vi "Main.vi"() -> ()   [LabVIEW 2018]
uses:
  LoadCellType.ctl
  MotorUnits.ctl
  <vilib>/Analysis/baseanly.llb/Mean (DBL).vi
  <vilib>/FPGAPlugInAG/myRIO-1900/niLvFpga_Open_myRIO-1900.vi
  <vilib>/rvi/interface/common/dynamic/niFpgaDynamicAddResources.vi
  <vilib>/FPGAPlugInAG/Dynamic/niLvFpga_Run_Dynamic.vi
  <vilib>/Utility/error.llb/Error Cluster From Error Code.vi
  <vilib>/rvi/errors/niLvFpgaAdjustHostInterfaceError.vi
  <vilib>/FPGAPlugInAG/Dynamic/niLvFpga_Abort_Dynamic.vi
  <vilib>/FPGAPlugInAG/Dynamic/niLvFpga_Close_Dynamic.vi
  <vilib>/rvi/interface/nirviOpenFPGA/nirviOpenFPGA.xnode
  FPGA Bitfiles/StandProgram_FPGATarget3_FPGARightReadout_3aa7no0+bKE.lvbitx
  FPGARightReadout.vi
  <vilib>/rvi/interface/nirviMethod/nirviMethod.xnode
  <vilib>/rvi/interface/nirviReadWriteControl/nirviReadWriteControl.xnode
  <vilib>/rvi/interface/nirviCloseFPGA/nirviCloseFPGA.xnode
  FPGA Bitfiles/StandProgram_FPGATarget_FPGACentreReadou_e9s0Pr-w3KU.lvbitx
  FPGACentreReadout.vi
  FPGA Bitfiles/StandProgram_FPGATarget2_FPGALeftReadout_XaESxvNjBQc.lvbitx
  FPGALeftReadout.vi
  NiFpgaLv.dll
  <vilib>/rvi/interface/Simulation/niFpgaSimulationCallBeginRW.vi
  <vilib>/Analysis/NI_AALBase.lvlib
  <userlib>/dxl_x86_c/dxl_x86_c.lvlib
panel:
  in  "Motor 2 Operating Mode":u16(ring)=5 caption="Operating Mode" items=["Please Select", "Current Control", "Velocity", "Position", "Extended Position", "Current-based Position Control"]
  out "Current Motor 1 Position":dbl(knob) scale=0.0..360.0
  in  "Motor 1 Operating Mode":u16(ring)=5 caption="Operating Mode" items=["Please Select", "Current Control", "Velocity", "Position", "Extended Position", "Current-based Position Control"]
  out "function return":i32
  in  "Left Stand":enum32{"Main", "Setup"}(tab)
  out "Left Motor Frequency":dbl caption="Motor Frequency"
  in  "Left PWM frequency":i16=50 caption="PWM Frequency (Hz)" min=50 max=400
  in  "Left PWM Switch":bool caption="PWM Switch"
  in  "Left PWM pulse width":u32=1000 caption="PWM Length (us)" min=1000 max=2000
  out "Left Current":dbl(knob) caption="Current (A)" scale=0.0..90.0
  out "Left Voltage":dbl(knob) caption="Voltage (V)" scale=0.0..60.0
  out "Left LC1":dbl(slide) scale=-10.0..10.0
  out "Left LC2":dbl(slide) scale=-5.0..5.0
  out "Left LC3":dbl(slide) scale=-5.0..5.0
  in  "Left Motor Units":T1 caption="Units" items=["RPM", "Hz"]
  out "Left LC1 Reading":i32 caption="Reading"
  in  "Left LC3 Calibrate":bool
  in  "Left LC3 Calibration Weight (kg)":dbl caption="Calibration Weight (kg)"
  in  "Left LC3 Type":T2 caption="Load Cell Type" items=["5kg", "10kg", "50kg"]
  out "Left LC3 zero point":i32 caption="Zero Point"
  in  "Left LC3 Tare":bool
  in  "Left LC2 Calibrate":bool
  in  "Left LC2 Calibration Weight (kg)":dbl caption="Calibration Weight (kg)"
  in  "Left LC2 Type":T2 caption="Load Cell Type" items=["5kg", "10kg", "50kg"]
  out "Left LC2 zero point":i32 caption="Zero Point"
  in  "Left LC2 Tare":bool
  in  "Left LC1 Calibrate 3":bool
  in  "Left LC1 Calibration Weight (kg)":dbl caption="Calibration Weight (kg)"
  in  "Left LC1 Type":T2=1 caption="Load Cell Type" items=["5kg", "10kg", "50kg"]
  out "Left LC1 zero point":i32=34722 caption="Zero Point"
  in  "Left LC1 Tare 3":bool
  out "Left LC3 Reading":i32 caption="Reading"
  out "Left LC2 Reading":i32 caption="Reading"
  in  "Left Resistance non-Vout (Ohms)":dbl=13.81
  in  "Left Resistance Vout (Ohms)":dbl=1.642
  out "Left Raw Load Cell Readings":cluster{"Data":i32, "Data 2":i32, "Data 3":i32}(graph) caption="Raw Load Cell Readings"
  out "Left LC3 Calibration Constant":dbl format="%#_13g"
  out "Left LC2 Calibration Constant":dbl format="%#_13g"
  out "Left LC1 Calibration Constant":dbl format="%#_13g"
  in  "Centre Stand":enum32{"Main", "Setup"}(tab)
  out "Right LC1":dbl(slide) scale=-10.0..10.0
  out "Left LC2":dbl(slide) scale=-10.0..10.0
  out "Centre LC3":dbl(slide) scale=-10.0..10.0
  out "Centre LC1 Reading":i32 caption="Reading"
  in  "Centre LC3 Calibrate":bool
  in  "Centre LC3 Calibration Weight (kg)":dbl caption="Calibration Weight (kg)"
  in  "Centre LC3 Type":T2=1 caption="Load Cell Type" items=["5kg", "10kg", "50kg"]
  out "Centre LC3 zero point":i32 caption="Zero Point"
  in  "Centre LC3 Tare":bool
  in  "Centre LC2 Calibrate":bool
  in  "Centre LC2 Calibration Weight (kg)":dbl caption="Calibration Weight (kg)"
  in  "Centre LC2 Type":T2=1 caption="Load Cell Type" items=["5kg", "10kg", "50kg"]
  out "Centre LC2 zero point":i32 caption="Zero Point"
  in  "Centre LC2 Tare":bool
  in  "Centre LC1 Calibrate":bool
  in  "Centre LC1 Calibration Weight (kg)":dbl caption="Calibration Weight (kg)"
  in  "Centre LC1 Type":T2=1 caption="Load Cell Type" items=["5kg", "10kg", "50kg"]
  out "Centre LC1 zero point":i32=34722 caption="Zero Point"
  in  "Centre LC1 Tare":bool
  out "Centre LC3 Reading":i32 caption="Reading"
  out "Centre LC2 Reading":i32 caption="Reading"
  out "Centre Raw Load Cell Readings":cluster{"Data":i32, "Data 2":i32, "Data 3":i32}(graph) caption="Raw Load Cell Readings"
  out "Centre LC3 Calibration Constant":dbl format="%#_13g"
  out "Centre LC2 Calibration Constant":dbl format="%#_13g"
  out "Centre LC1 Calibration Constant":dbl format="%#_13g"
  out "StopLoops":bool
  in  "Program Stop":bool
  out "Current Motor 2 Position":dbl(knob) scale=0.0..360.0
  in  "Target Motor 2 Position":dbl(knob) scale=0.0..360.0
  in  "Target Motor 1 Position":dbl(knob) scale=0.0..360.0
  in  "Right Stand":enum32{"Main", "Setup"}(tab)
  out "Right Motor Frequency":dbl caption="Motor Frequency"
  in  "Right PWM frequency":i16=50 caption="PWM Frequency (Hz)" min=50 max=400
  in  "Right PWM Switch":bool caption="PWM Switch"
  in  "Right PWM pulse width":u32=1000 caption="PWM Length (us)" min=1000 max=2000
  out "Right Current":dbl(knob) caption="Current (A)" scale=0.0..90.0
  out "Right Voltage":dbl(knob) caption="Voltage (V)" scale=0.0..60.0
  out "Right LC1":dbl(slide) scale=-10.0..10.0
  out "Right LC2":dbl(slide) scale=-5.0..5.0
  out "Right LC3":dbl(slide) scale=-5.0..5.0
  in  "Right Motor Units":T1 caption="Units" items=["RPM", "Hz"]
  out "Right LC1 Reading":i32 caption="Reading"
  in  "Right LC3 Calibrate":bool
  in  "Right LC3 Calibration Weight (kg)":dbl caption="Calibration Weight (kg)"
  in  "Right LC3 Type":T2 caption="Load Cell Type" items=["5kg", "10kg", "50kg"]
  out "Right LC3 zero point":i32 caption="Zero Point"
  in  "Right LC3 Tare":bool
  in  "Right LC2 Calibrate":bool
  in  "Right LC2 Calibration Weight (kg)":dbl caption="Calibration Weight (kg)"
  in  "Right LC2 Type":T2 caption="Load Cell Type" items=["5kg", "10kg", "50kg"]
  out "Right LC2 zero point":i32 caption="Zero Point"
  in  "Right LC2 Tare":bool
  in  "Right LC1 Calibrate":bool
  in  "Right LC1 Calibration Weight (kg)":dbl caption="Calibration Weight (kg)"
  in  "Right LC1 Type":T2=1 caption="Load Cell Type" items=["5kg", "10kg", "50kg"]
  out "Right LC1 zero point":i32=34722 caption="Zero Point"
  in  "Right LC1 Tare":bool
  out "Right LC3 Reading":i32 caption="Reading"
  out "Right LC2 Reading":i32 caption="Reading"
  in  "Right Resistance non-Vout (Ohms)":dbl=13.81
  in  "Right Resistance Vout (Ohms)":dbl=1.642
  out "Right Raw Load Cell Readings":cluster{"Data":i32, "Data 2":i32, "Data 3":i32}(graph) caption="Raw Load Cell Readings"
  out "Right LC1 Calibration Constant":dbl format="%#_13g"
  out "Right LC2 Calibration Constant":dbl format="%#_13g"
  out "Right LC3 Calibration Constant":dbl format="%#_13g"
  # "Centre Stand"
  # "Left Stand"
  # "Right Stand"
  # "Motor 1 Control"
  # "Motor 2 Control"
  # "Current position"
  # "Current position"
  # "Set position"
  # "Set position"
  # "Load Cell 1"
  # "Load Cell 2"
  # "Load Cell 3"
  # "Voltmeter"
  # "Load Cell 1"
  # "Load Cell 2"
  # "Load Cell 3"
  # "Load Cell 1"
  # "Load Cell 2"
  # "Load Cell 3"
  # "Voltmeter"
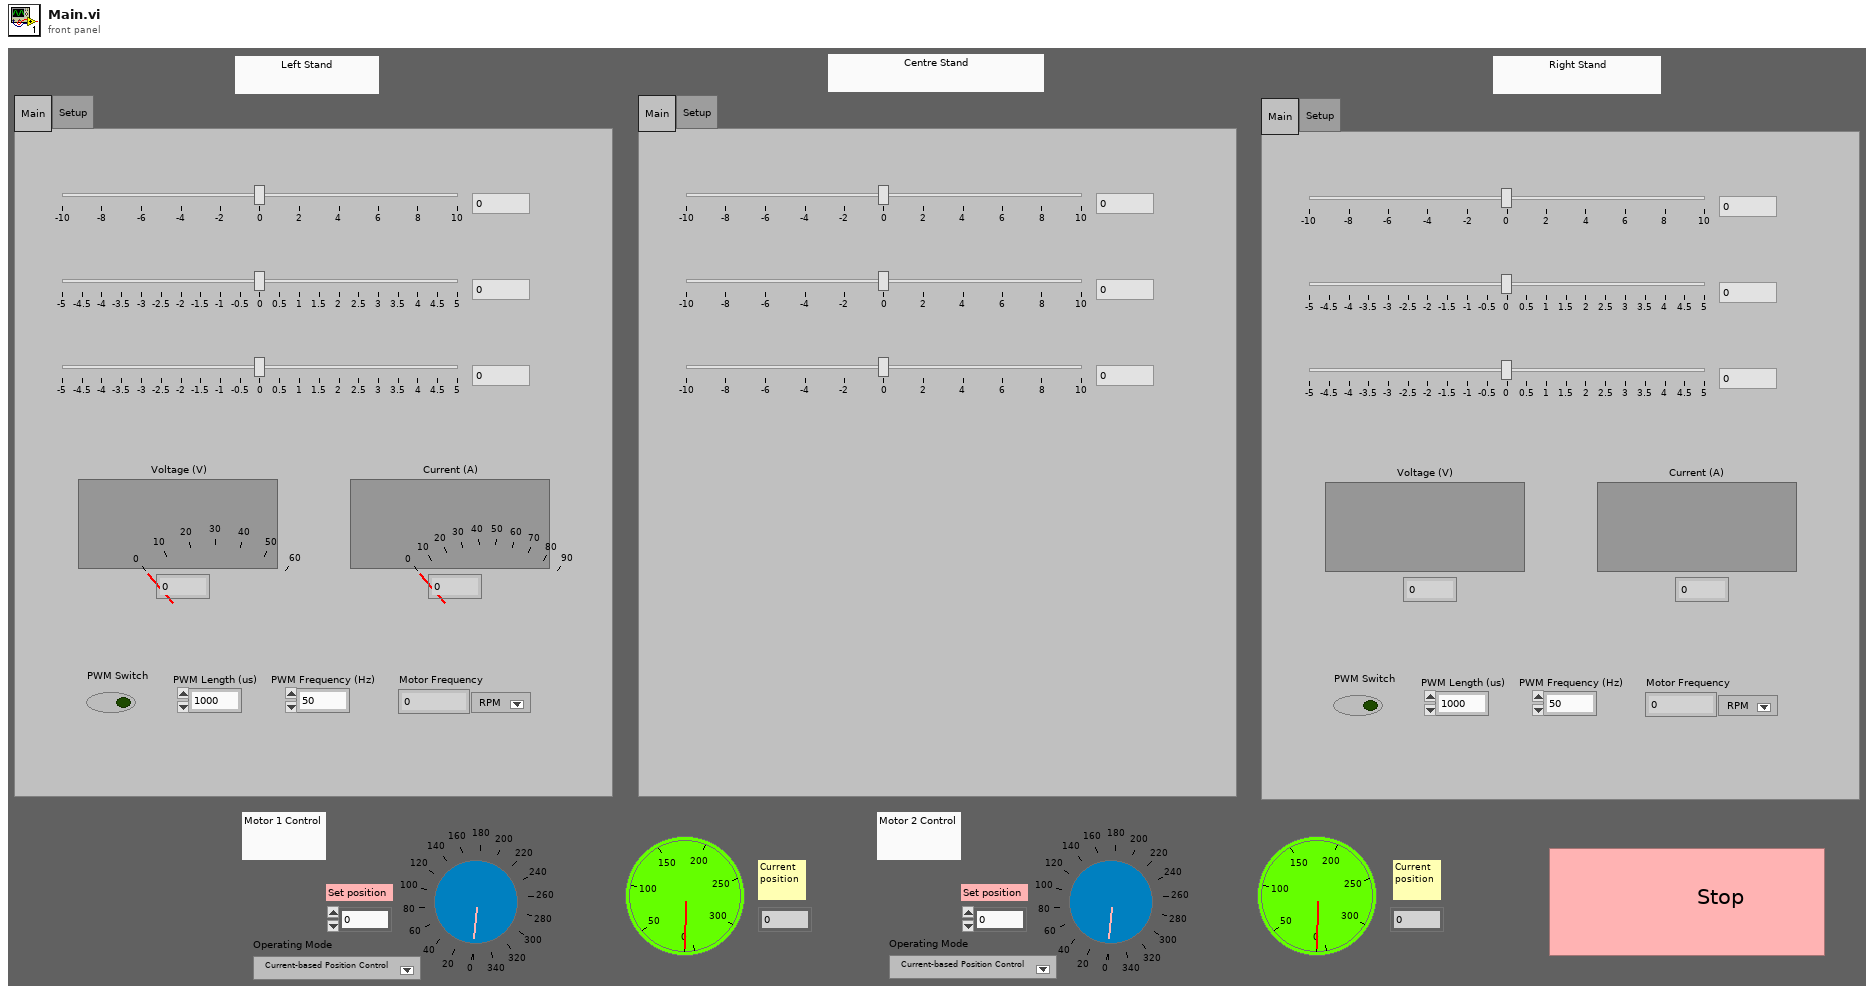
[diagram p1: front panel]
types:
  T1 = typedef "MotorUnits.ctl" = u16
  T2 = typedef "LoadCellType.ctl" = u16
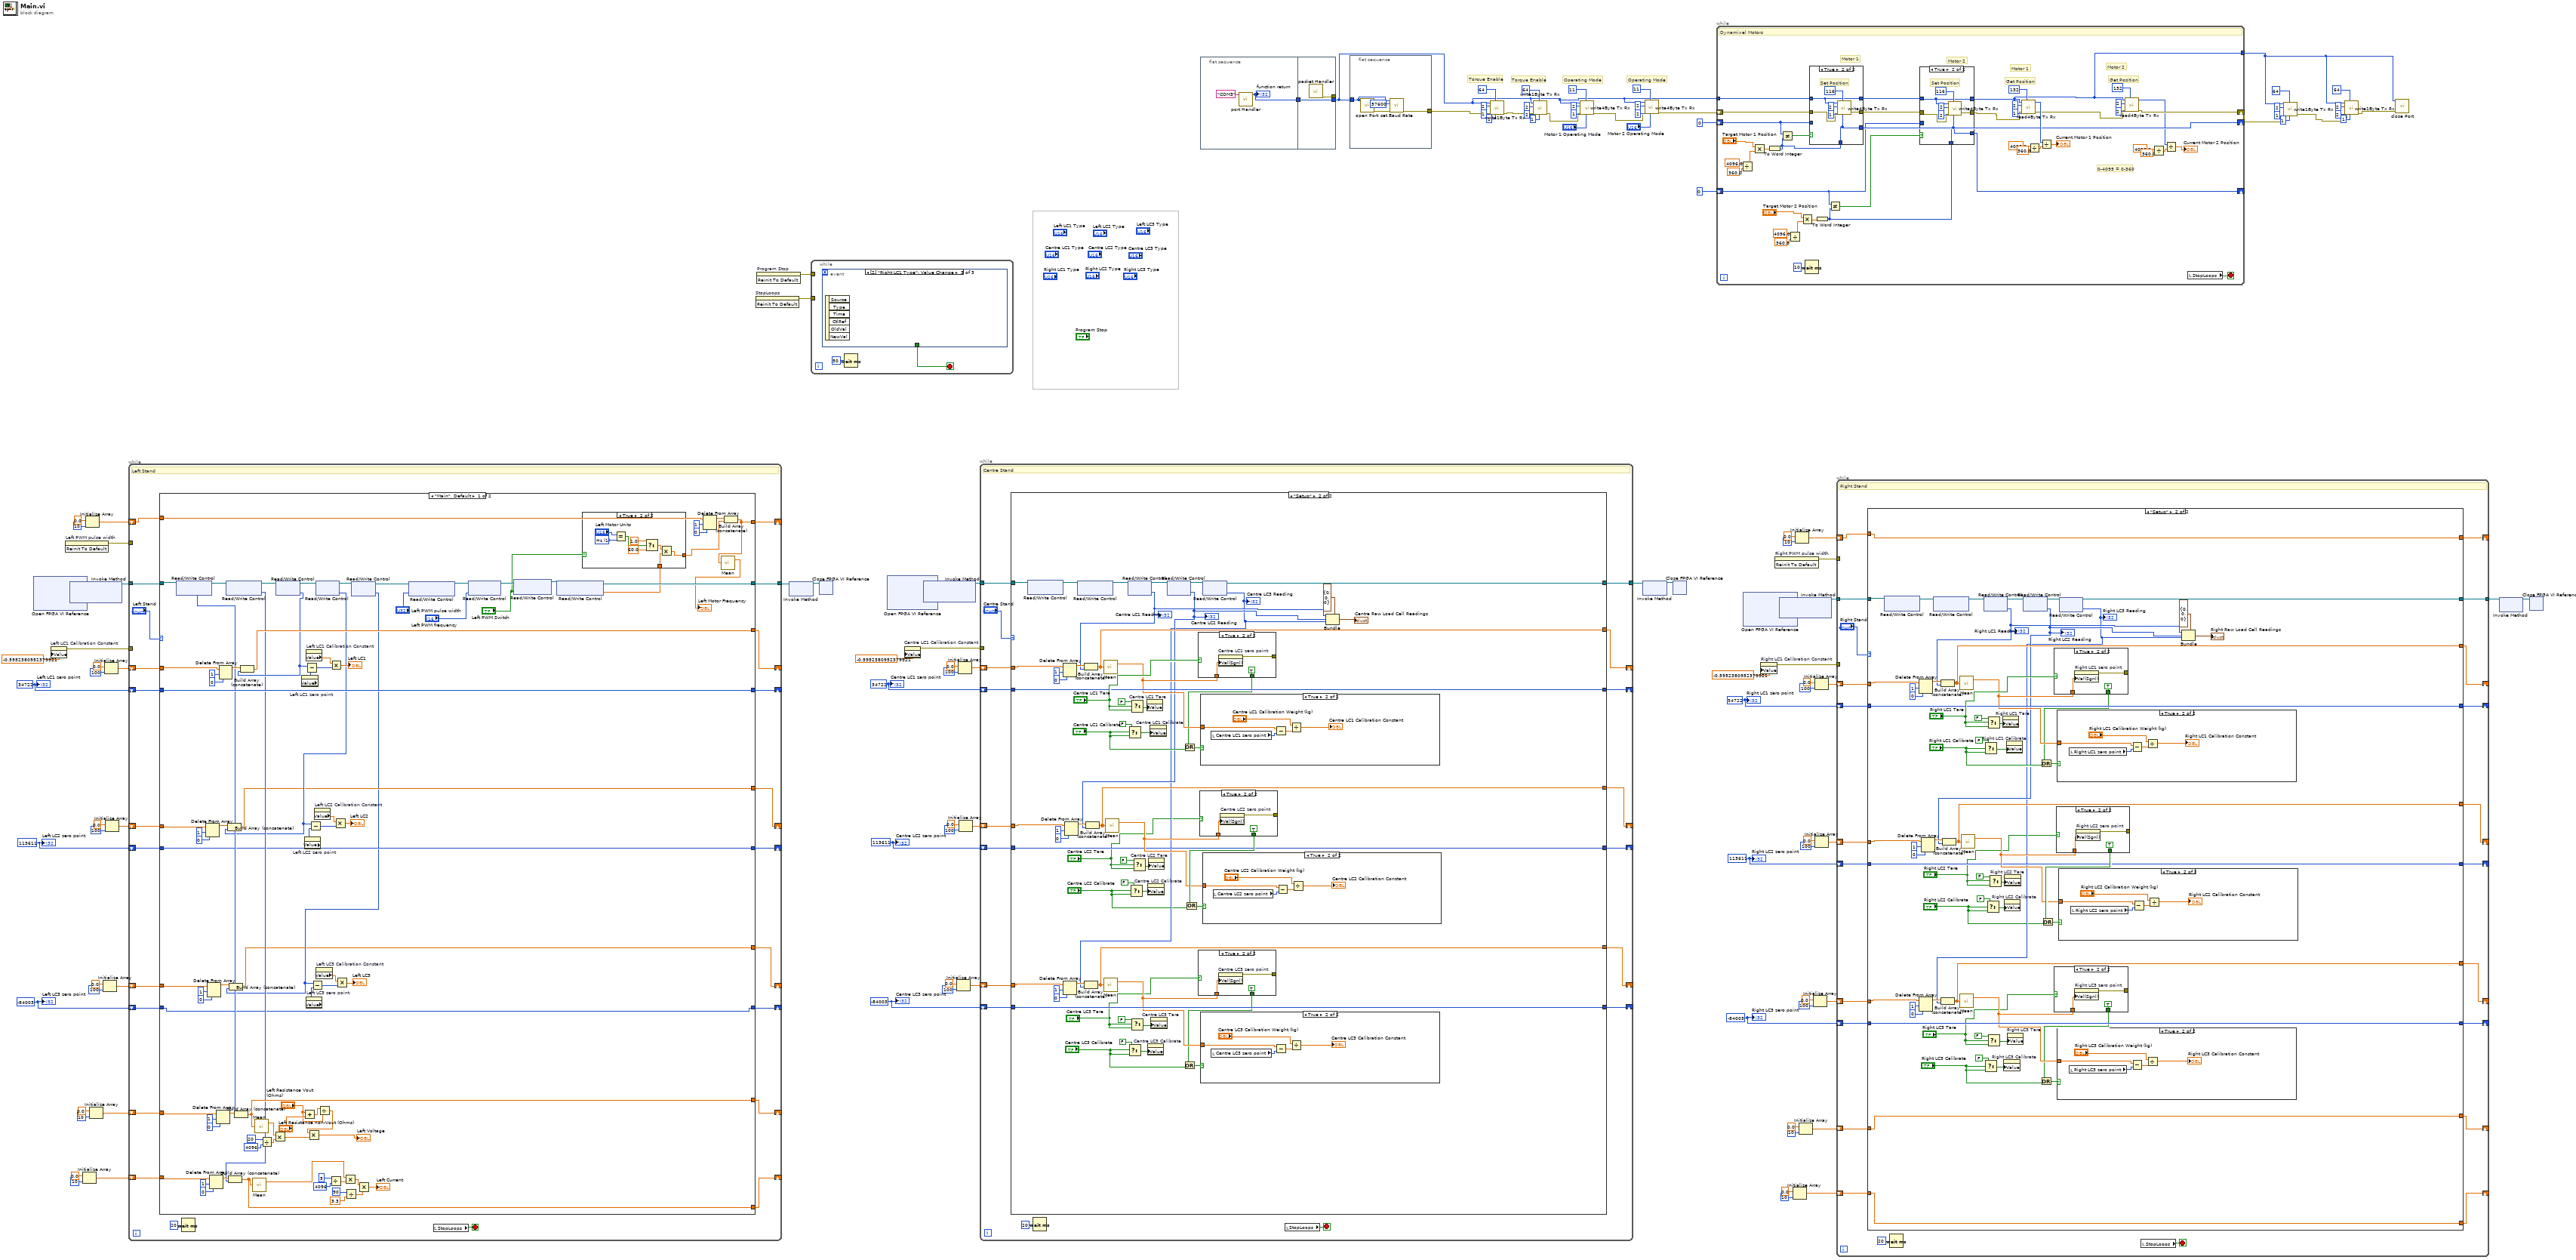
[diagram p0: block diagram]
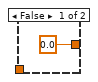
[diagram p4: hidden frame]
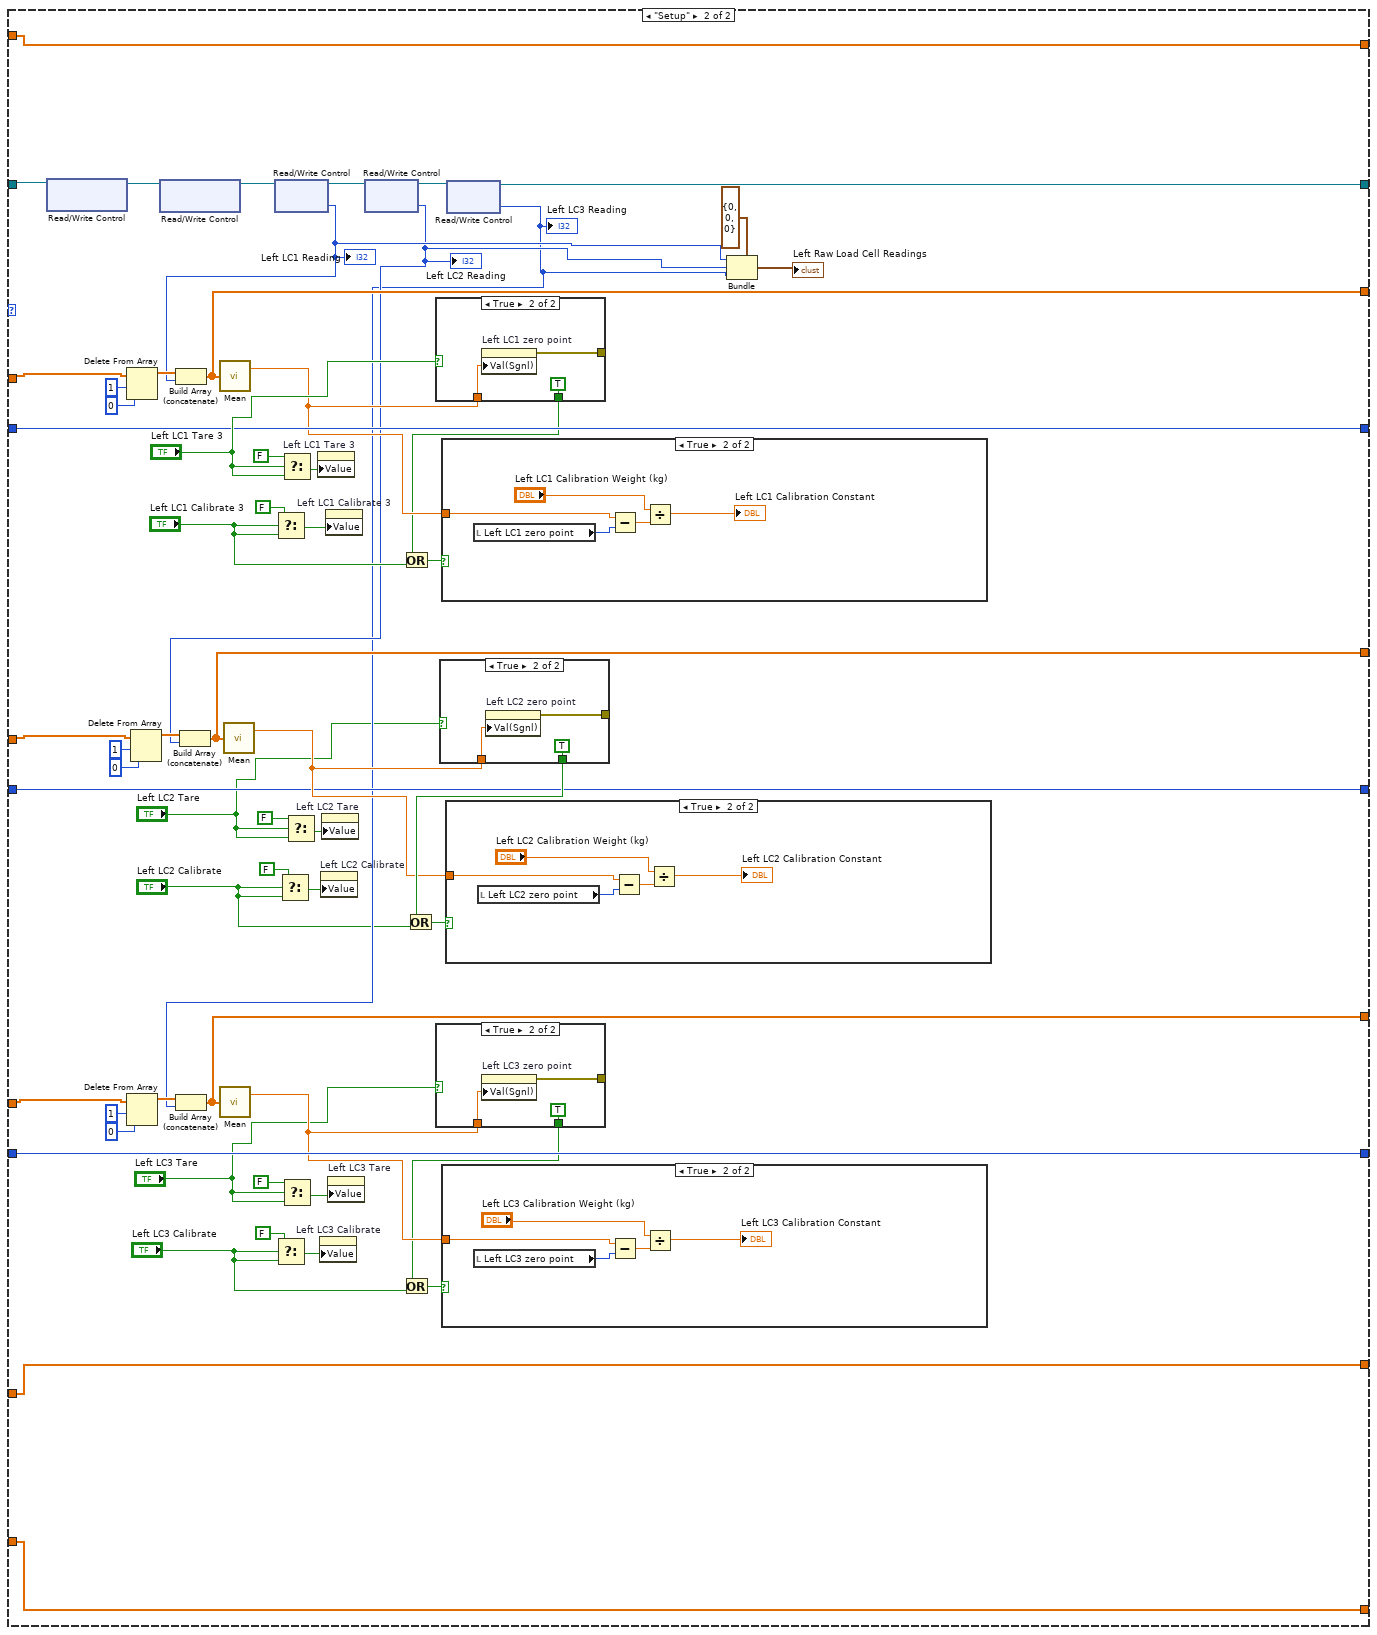
[diagram p5: hidden frame]
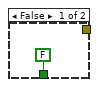
[diagram p7: hidden frame]
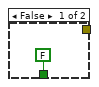
[diagram p9: hidden frame]
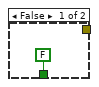
[diagram p11: hidden frame]
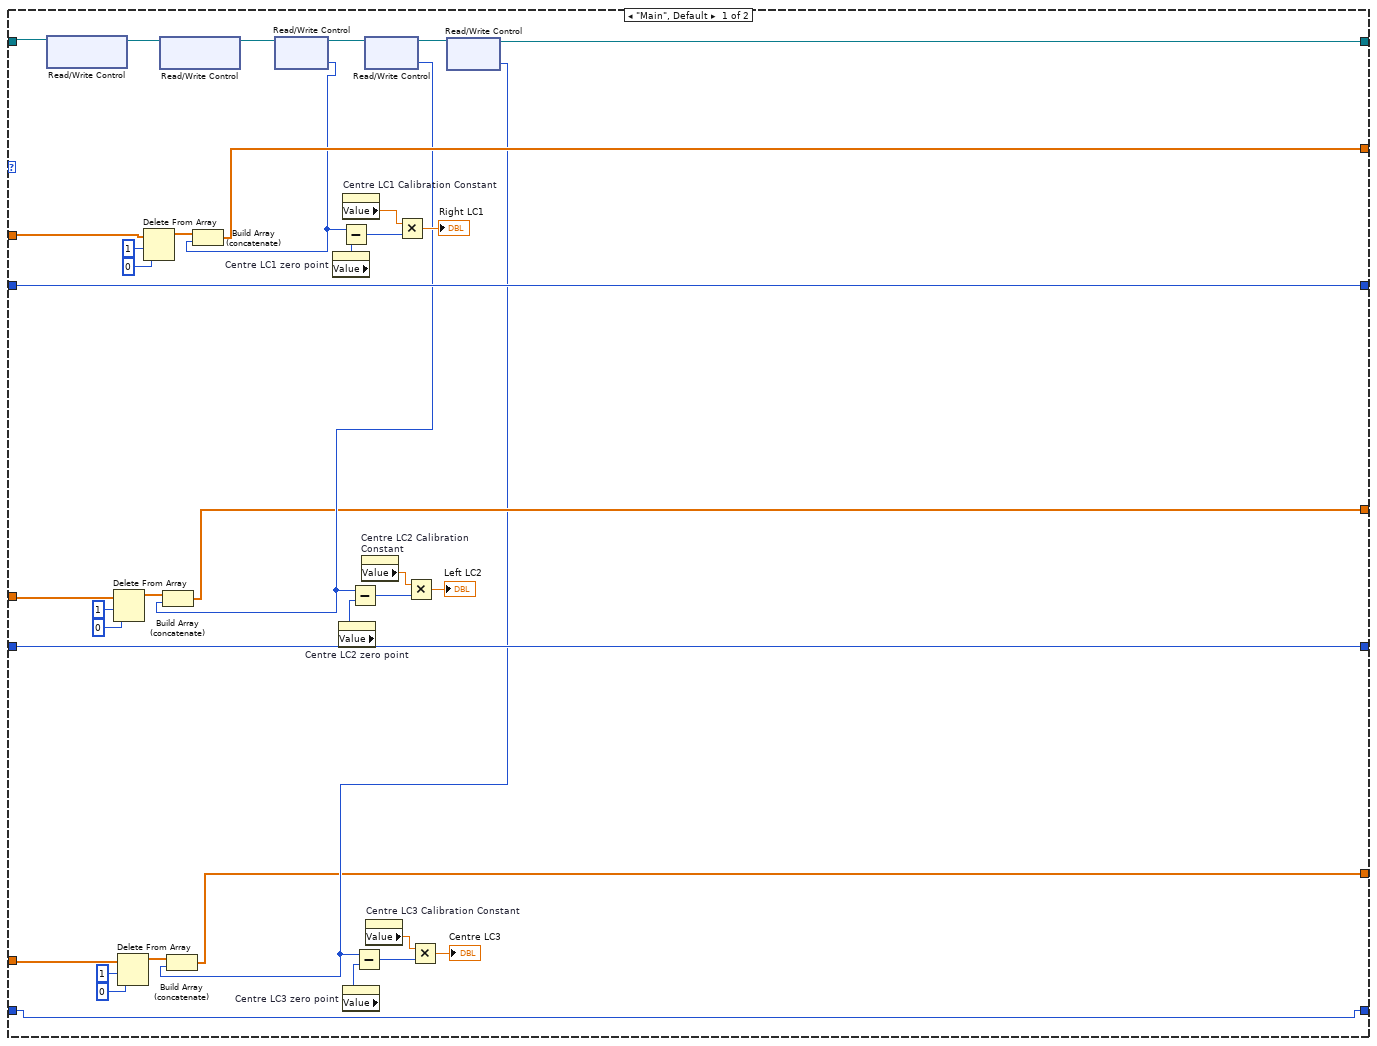
[diagram p12: hidden frame]
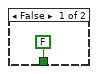
[diagram p14: hidden frame]
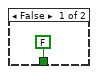
[diagram p16: hidden frame]
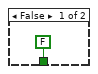
[diagram p18: hidden frame]
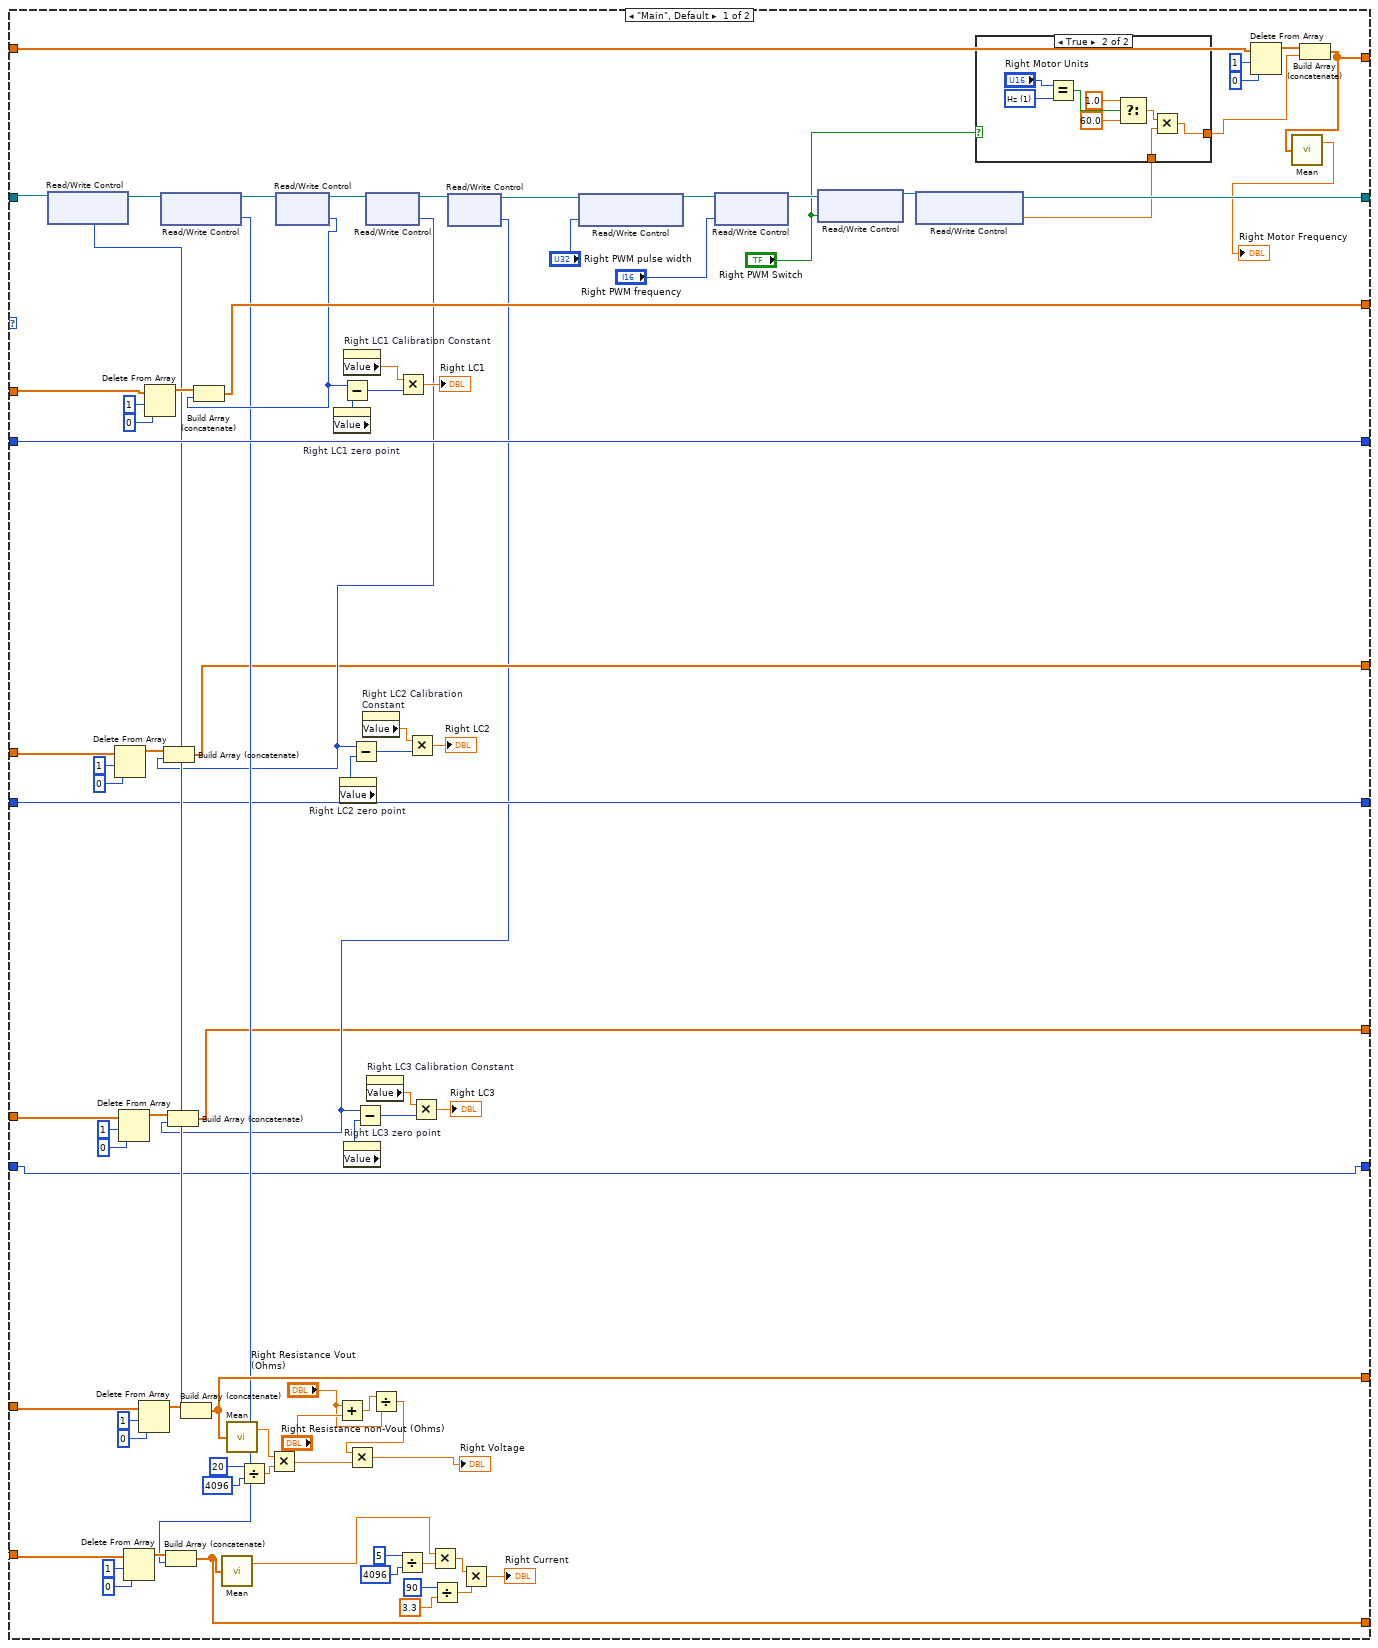
[diagram p19: hidden frame]
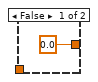
[diagram p20: hidden frame]
diagram:
  w38 = -84003 ("Right LC1 zero point")
  w42 = 113611 ("Right LC1 zero point")
  w51 = 34722 ("Right LC1 zero point")
  w82 = -84003 ("Right LC1 zero point")
  w78 = 113611 ("Right LC1 zero point")
  w72 = 34722 ("Right LC1 zero point")
  w84 = -84003 ("Right LC1 zero point")
  w88 = 113611 ("Right LC1 zero point")
  w97 = 34722 ("Right LC1 zero point")
  # "Operating Mode"
  # "Torque Enable"
  # "Operating Mode"
  # "Torque Enable"
  n1 = xnode "Open FPGA VI Reference"() -> ("FPGA VI Reference Out"=w65:refnum<k20>)  [unwired: 2 in, 1 out]
  n2 = property on="Left LC1 Calibration Constant" class="DigNum (strict)"("Value"=-0.5952380952379921 ("Right LC1 Calibration Constant")) -> (error out=w50:errorcluster)  [unwired: 2 in, 1 out]
  n3 = invoke on="Left PWM pulse width" class="DigNum (strict)" method="Reinit To Default"() -> (error out=w55:errorcluster)  [unwired: 3 in, 2 out]
  n4 = xnode "Invoke Method"("FPGA VI Reference In"=w65) -> ("FPGA VI Reference Out"=w64:refnum<k20>)  [unwired: 2 in, 1 out]
  n5 = Initialize Array(0.0 ("element"), 10 ("dimension size")) -> (w52:dbl[])
  n6 = Initialize Array(0.0 ("element"), 10 ("dimension size")) -> (w48:dbl[])
  n7 = Initialize Array(0.0 ("element"), 10 ("dimension size")) -> (w58:dbl[])
  n8 = Initialize Array(0.0 ("element"), 100 ("dimension size")) -> (w39:dbl[])
  n9 = Initialize Array(0.0 ("element"), 100 ("dimension size")) -> (w59:dbl[])
  n10 = Initialize Array(0.0 ("element"), 100 ("dimension size")) -> (w45:dbl[])
  n11 = while {
    tunnel: w64 -> [w135]
    tunnel: [w134] -> w62
    shift-right: [w130] -> _
    shift-left: w51 -> [w132]
    shift-right: [w129] -> _
    shift-left: w59 -> [w131]
    shift-right: [w126] -> _
    shift-left: w58 -> [w127]
    tunnel: w55 -> [_]
    shift-right: [w124] -> _
    shift-left: w52 -> [w125]
    tunnel: w50 -> [_]
    shift-right: [w122] -> _
    shift-left: w48 -> [w123]
    shift-right: [w118] -> _
    shift-left: w42 -> [w120]
    shift-right: [w119] -> _
    shift-left: w45 -> [w121]
    shift-right: [w117] -> _
    shift-left: w38 -> [w115]
    shift-right: [w116] -> _
    shift-left: w39 -> [w114]
    stop <- w136 stop-if-true
    # "Left Stand"
    n12 = case shown="\"Main\", Default" "Left Stand" {
      tunnel: w135 -> [w221 w289]
      tunnel: [w170 w284] -> w134
      tunnel: w132 -> [w211 w275]
      tunnel: w131 -> [w213 w278]
      tunnel: [w211 w275] -> w130
      tunnel: [w212 w276] -> w129
      tunnel: w127 -> [w196 w268]
      tunnel: [w195 w268] -> w126
      tunnel: w125 -> [w178 w267]
      tunnel: [w173 w267] -> w124
      tunnel: w123 -> [w165 w263]
      tunnel: [w162 w263] -> w122
      tunnel: w120 -> [w151 w251]
      tunnel: w121 -> [w157 w254]
      tunnel: [w152 w252] -> w119
      tunnel: [w151 w251] -> w118
      tunnel: w115 -> [w144 w250]
      tunnel: w114 -> [w143 w248]
      tunnel: [w140 w249] -> w116
      tunnel: [w144 w250] -> w117
      frame "Main", Default {
        n13 = xnode "Read/Write Control"("FPGA VI Reference In"=w221) -> ("FPGA VI Reference Out"=w220:refnum<k20>, "RawVoltage"=w193:i16)  [unwired: 1 in, 1 out]
        n14 = Delete From Array(array=w157, length=1, index=0) -> (array with subset deleted=w158:dbl[])  [unwired: 1 out]
        n15 = Delete From Array(array=w143, length=1, index=0) -> (array with subset deleted=w148:dbl[])  [unwired: 1 out]
        n16 = Delete From Array(array=w178, length=1, index=0) -> (array with subset deleted=w177:dbl[])  [unwired: 1 out]
        n17 = Delete From Array(array=w196, length=1, index=0) -> (array with subset deleted=w202:dbl[])  [unwired: 1 out]
        n18 = Delete From Array(array=w213, length=1, index=0) -> (array with subset deleted=w216:dbl[])  [unwired: 1 out]
        n19 = xnode "Read/Write Control"("FPGA VI Reference In"=w220) -> ("FPGA VI Reference Out"=w219:refnum<k20>, "RawCurrent"=w174:u16)  [unwired: 1 in, 1 out]
        n20 = Build Array (concatenate)(w177, w174) -> (w173:dbl[])
        n21 = Build Array (concatenate)(w202, w193) -> (w195:dbl[])
        n22 = call-poly <vilib>:"Mean.vi"("X"=w173) -> ("mean"=w172:dbl)  [unwired: 1 out]
        n23 = call-poly <vilib>:"Mean.vi"("X"=w195) -> ("mean"=w200:dbl)  [unwired: 1 out]
        n24 = Divide(x=i16 20, y=i16 4096) -> (x/y=w201:dbl)
        n25 = Multiply(x=w200, y=w201) -> (x*y=w198:dbl)
        n26 = xnode "Read/Write Control"("FPGA VI Reference In"=w219) -> ("FPGA VI Reference Out"=w218:refnum<k20>, "Data"=w207:i32)  [unwired: 1 in, 1 out]
        n27 = Build Array (concatenate)(w216, w207) -> (w212:dbl[])
        n28 = property on="Left LC1 zero point" class="DigNum (strict)"() -> ("Value"=w208:i32)  [unwired: 2 in, 2 out]
        n29 = Add(x="Left Resistance Vout (Ohms)", y="Left Resistance non-Vout (Ohms)") -> (x+y=w192:dbl)
        n30 = property on="Left LC2 zero point" class="DigNum (strict)"() -> ("Value"=w154:i32)  [unwired: 2 in, 2 out]
        n31 = Subtract(x=w207, y=w208) -> (x-y=w209:i32)
        n32 = property on="Left LC1 Calibration Constant" class="DigNum (strict)"() -> ("Value"=w210:dbl)  [unwired: 2 in, 2 out]
        n33 = property on="Left LC3 zero point" class="DigNum (strict)"() -> ("Value"=w150:i32)  [unwired: 2 in, 2 out]
        n34 = property on="Left LC2 Calibration Constant" class="DigNum (strict)"() -> ("Value"=w155:dbl)  [unwired: 2 in, 2 out]
        n35 = xnode "Read/Write Control"("FPGA VI Reference In"=w218) -> ("FPGA VI Reference Out"=w217:refnum<k20>, "Data 2"=w153:i32)  [unwired: 1 in, 1 out]
        n36 = Build Array (concatenate)(w158, w153) -> (w152:dbl[])
        n37 = Subtract(x=w153, y=w154) -> (x-y=w161:i32)
        n38 = property on="Left LC3 Calibration Constant" class="DigNum (strict)"() -> ("Value"=w149:dbl)  [unwired: 2 in, 2 out]
        n39 = Divide(x=w192, y="Left Resistance Vout (Ohms)") -> (x/y=w197:dbl)
        n40 = Multiply(x=w197, y=w198) -> (x*y=→"Left Voltage":dbl)
        n41 = Divide(x=i16 5, y=i16 4096) -> (x/y=w188:dbl)
        n42 = Multiply(x=w210, y=w209) -> (x*y=→"Left LC1":dbl)
        n43 = Multiply(x=w155, y=w161) -> (x*y=→"Left LC2":dbl)
        n44 = Multiply(x=w172, y=w188) -> (x*y=w180:dbl)
        n45 = Divide(x=i16 90 ("y"), y=3.3 ("x")) -> (x/y=w187:dbl)
        n46 = xnode "Read/Write Control"("FPGA VI Reference In"=w217) -> ("FPGA VI Reference Out"=w186:refnum<k20>, "Data 3"=w141:i32)  [unwired: 1 in, 1 out]
        n47 = Build Array (concatenate)(w148, w141) -> (w140:dbl[])
        n48 = Subtract(x=w141, y=w150) -> (x-y=w145:i32)
        n49 = Multiply(x=w149, y=w145) -> (x*y=→"Left LC3":dbl)
        n50 = Multiply(x=w180, y=w187) -> (x*y=→"Left Current":dbl)
        n51 = xnode "Read/Write Control"("FPGA VI Reference In"=w186, "Pulse Width (us)"="Left PWM pulse width") -> ("FPGA VI Reference Out"=w185:refnum<k20>)  [unwired: 1 in, 1 out]
        n52 = xnode "Read/Write Control"("FPGA VI Reference In"=w185, "Frequency"="Left PWM frequency") -> ("FPGA VI Reference Out"=w184:refnum<k20>)  [unwired: 1 in, 1 out]
        n53 = xnode "Read/Write Control"("FPGA VI Reference In"=w184, "PWM Switch"="Left PWM Switch") -> ("FPGA VI Reference Out"=w183:refnum<k20>)  [unwired: 1 in, 1 out]
        n54 = xnode "Read/Write Control"("FPGA VI Reference In"=w183) -> ("FPGA VI Reference Out"=w170:refnum<k20>, "Rotor Speed (Hz)"=w169:sgl)  [unwired: 1 in, 1 out]
        n55 = case shown="True" "Left PWM Switch" {
          tunnel: [0.0 ("Motor Frequency") w224] -> w164
          tunnel: w169 -> [_ w223]
          frame False {
          }
          frame True {
            w230 = T1 1 items=["RPM", "Hz"] ("Right Motor Units")
            n56 = Equal?(x="Left Motor Units", y=w230) -> (x = y?=w229:bool)
            n57 = Select(t=1.0, s=w229, f=60.0) -> (s? t:f=w225:dbl)
            n58 = Multiply(x=w225, y=w223) -> (x*y=w224:dbl)
          }
        }
        n59 = Delete From Array(array=w165, length=1, index=0) -> (array with subset deleted=w166:dbl[])  [unwired: 1 out]
        n60 = Build Array (concatenate)(w166, w164) -> (w162:dbl[])
        n61 = call-poly <vilib>:"Mean.vi"("X"=w162) -> ("mean"=→"Left Motor Frequency":dbl)  [unwired: 1 out]
      }
      frame "Setup" {
        n62 = xnode "Read/Write Control"("FPGA VI Reference In"=w289) -> ("FPGA VI Reference Out"=w288:refnum<k20>)  [unwired: 1 in, 2 out]
        n63 = Delete From Array(array=w278, length=1, index=0) -> (array with subset deleted=w277:dbl[])  [unwired: 1 out]
        n64 = Delete From Array(array=w248, length=1, index=0) -> (array with subset deleted=w244:dbl[])  [unwired: 1 out]
        n65 = Delete From Array(array=w254, length=1, index=0) -> (array with subset deleted=w258:dbl[])  [unwired: 1 out]
        n66 = xnode "Read/Write Control"("FPGA VI Reference In"=w288) -> ("FPGA VI Reference Out"=w287:refnum<k20>)  [unwired: 1 in, 2 out]
        n67 = xnode "Read/Write Control"("FPGA VI Reference In"=w287) -> ("FPGA VI Reference Out"=w286:refnum<k20>, "Data"=w266:i32)  [unwired: 1 in, 1 out]
        "Left LC1 Reading" <- w266
        n68 = Build Array (concatenate)(w277, w266) -> (w276:dbl[])
        n69 = call-poly <vilib>:"Mean.vi"("X"=w276) -> ("mean"=w273:dbl)  [unwired: 1 out]
        n70 = Select(t=FALSE, s="Left LC1 Calibrate 3", f="Left LC1 Calibrate 3") -> (s? t:f=w271:bool)
        n71 = Select(t=FALSE, s="Left LC3 Calibrate", f="Left LC3 Calibrate") -> (s? t:f=w232:bool)
        n72 = Select(t=FALSE, s="Left LC2 Calibrate", f="Left LC2 Calibrate") -> (s? t:f=w235:bool)
        n73 = Select(t=FALSE, s="Left LC1 Tare 3", f="Left LC1 Tare 3") -> (s? t:f=w283:bool)
        n74 = Select(t=FALSE, s="Left LC3 Tare", f="Left LC3 Tare") -> (s? t:f=w231:bool)
        n75 = Select(t=FALSE, s="Left LC2 Tare", f="Left LC2 Tare") -> (s? t:f=w237:bool)
        n76 = property on="Left LC1 Tare 3" class="Bool (strict)"("Value"=w283) -> ()  [unwired: 2 in, 2 out]
        n77 = property on="Left LC3 Calibrate" class="Bool (strict)"("Value"=w232) -> ()  [unwired: 2 in, 2 out]
        n78 = property on="Left LC2 Calibrate" class="Bool (strict)"("Value"=w235) -> ()  [unwired: 2 in, 2 out]
        n79 = property on="Left LC2 Tare" class="Bool (strict)"("Value"=w237) -> ()  [unwired: 2 in, 2 out]
        n80 = property on="Left LC1 Calibrate 3" class="Bool (strict)"("Value"=w271) -> ()  [unwired: 2 in, 2 out]
        n81 = property on="Left LC3 Tare" class="Bool (strict)"("Value"=w231) -> ()  [unwired: 2 in, 2 out]
        n82 = xnode "Read/Write Control"("FPGA VI Reference In"=w286) -> ("FPGA VI Reference Out"=w285:refnum<k20>, "Data 2"=w253:i32)  [unwired: 1 in, 1 out]
        "Left LC2 Reading" <- w253
        n83 = Build Array (concatenate)(w258, w253) -> (w252:dbl[])
        n84 = call-poly <vilib>:"Mean.vi"("X"=w252) -> ("mean"=w260:dbl)  [unwired: 1 out]
        n85 = case shown="True" "Left LC1 Tare 3" {
          tunnel: w273 -> [_ w316]
          tunnel: [FALSE TRUE] -> w270
          tunnel: [_ w314] -> _
          frame False {
          }
          frame True {
            n86 = property on="Left LC1 zero point" class="DigNum (strict)"("Val(Sgnl)"=w316) -> (error out=w314:errorcluster)  [unwired: 2 in, 1 out]
          }
        }
        n87 = Or(x=w270, y="Left LC1 Calibrate 3") -> (x .or. y?=w272:bool)
        n88 = case shown="True" "Left LC2 Tare" {
          tunnel: w260 -> [_ w307]
          tunnel: [FALSE TRUE] -> w262
          tunnel: [_ w305] -> _
          frame False {
          }
          frame True {
            n89 = property on="Left LC2 zero point" class="DigNum (strict)"("Val(Sgnl)"=w307) -> (error out=w305:errorcluster)  [unwired: 2 in, 1 out]
          }
        }
        n90 = Or(x=w262, y="Left LC2 Calibrate") -> (x .or. y?=w261:bool)
        n91 = case shown="True" w272 {
          tunnel: w273 -> [_ w312]
          frame False {
          }
          frame True {
            n92 = local read "Left LC1 zero point"() -> (w311:i32)
            n93 = Subtract(x=w312, y=w311) -> (x-y=w310:dbl)
            n94 = Divide(x="Left LC1 Calibration Weight (kg)", y=w310) -> (x/y=→"Left LC1 Calibration Constant":dbl)
          }
        }
        n95 = case shown="True" w261 {
          tunnel: w260 -> [_ w303]
          frame False {
          }
          frame True {
            n96 = local read "Left LC2 zero point"() -> (w302:i32)
            n97 = Subtract(x=w303, y=w302) -> (x-y=w301:dbl)
            n98 = Divide(x="Left LC2 Calibration Weight (kg)", y=w301) -> (x/y=→"Left LC2 Calibration Constant":dbl)
          }
        }
        n99 = xnode "Read/Write Control"("FPGA VI Reference In"=w285) -> ("FPGA VI Reference Out"=w284:refnum<k20>, "Data 3"=w239:i32)  [unwired: 1 in, 1 out]
        "Left LC3 Reading" <- w239
        n100 = Build Array (concatenate)(w244, w239) -> (w249:dbl[])
        n101 = call-poly <vilib>:"Mean.vi"("X"=w249) -> ("mean"=w242:dbl)  [unwired: 1 out]
        n102 = case shown="True" "Left LC3 Tare" {
          tunnel: w242 -> [_ w298]
          tunnel: [FALSE TRUE] -> w240
          tunnel: [_ w296] -> _
          frame False {
          }
          frame True {
            n103 = property on="Left LC3 zero point" class="DigNum (strict)"("Val(Sgnl)"=w298) -> (error out=w296:errorcluster)  [unwired: 2 in, 1 out]
          }
        }
        n104 = Or(x=w240, y="Left LC3 Calibrate") -> (x .or. y?=w241:bool)
        n105 = case shown="True" w241 {
          tunnel: w242 -> [_ w294]
          frame False {
          }
          frame True {
            n106 = local read "Left LC3 zero point"() -> (w293:i32)
            n107 = Subtract(x=w294, y=w293) -> (x-y=w292:dbl)
            n108 = Divide(x="Left LC3 Calibration Weight (kg)", y=w292) -> (x/y=→"Left LC3 Calibration Constant":dbl)
          }
        }
        n109 = Bundle(cluster=cluster{"Data":i32, "Data 2":i32, "Data 3":i32} {"Data"=0, "Data 2"=0, "Data 3"=0}, "Data"=w266, "Data 2"=w253, "Data 3"=w239) -> (→"Left Raw Load Cell Readings":cluster{"Data":i32, "Data 2":i32, "Data 3":i32})
      }
    }
    n110 = Wait (ms)(milliseconds to wait=u32 20) -> ()  [unwired: 1 out]
    n111 = local read "StopLoops"() -> (w136:bool)
  }
  n112 = invoke on="StopLoops" class="Bool (strict)" method="Reinit To Default"() -> (error out=w112:errorcluster)  [unwired: 3 in, 2 out]
  n113 = invoke on="Program Stop" class="Bool (strict)" method="Reinit To Default"() -> (error out=w113:errorcluster)  [unwired: 3 in, 2 out]
  n114 = xnode "Invoke Method"("FPGA VI Reference In"=w62) -> ("FPGA VI Reference Out"=w63:refnum<k20>)  [unwired: 1 in, 1 out]
  n115 = while {
    tunnel: w113 -> [_]
    tunnel: w112 -> [_]
    stop <- w317 stop-if-true
    n116 = event shown="[2] \"Right LC1 Type\": Value Change" {
      selector: _ -> [_ _ _]
      dyn-events: _ -> [_ _ _]
      timeout: _ -> [_ _ _]
      tunnel: [_ w319 _] -> w317
      event Timeout {
        n117 = event-data() -> ()  [unwired: 1 in, 3 out]
      }
      event "Program Stop": Value Change {
        w319 = TRUE
        n118 = event-data() -> ()  [unwired: 1 in, 6 out]
        "StopLoops" <- w319
      }
      event Value Change {
        n119 = event-data() -> ()  [unwired: 1 in, 6 out]
      }
    }
    n120 = Wait (ms)(milliseconds to wait=u32 50) -> ()  [unwired: 1 out]
  }
  n121 = xnode "Close FPGA VI Reference"("FPGA VI Reference In"=w63) -> ()  [unwired: 1 in, 1 out]
  n122 = xnode "Open FPGA VI Reference"() -> ("FPGA VI Reference Out"=w66:refnum<k20>)  [unwired: 2 in, 1 out]
  n123 = property on="Centre LC1 Calibration Constant" class="DigNum (strict)"("Value"=-0.5952380952379921 ("Right LC1 Calibration Constant")) -> (error out=w73:errorcluster)  [unwired: 2 in, 1 out]
  n124 = xnode "Invoke Method"("FPGA VI Reference In"=w66) -> ("FPGA VI Reference Out"=w67:refnum<k20>)  [unwired: 2 in, 1 out]
  n125 = Initialize Array(0.0 ("element"), 100 ("dimension size")) -> (w81:dbl[])
  n126 = Initialize Array(0.0 ("element"), 100 ("dimension size")) -> (w71:dbl[])
  n127 = Initialize Array(0.0 ("element"), 100 ("dimension size")) -> (w75:dbl[])
  n128 = while {
    tunnel: w67 -> [w335]
    tunnel: [w334] -> w68
    shift-right: [w330] -> _
    shift-left: w72 -> [w332]
    shift-right: [w329] -> _
    shift-left: w71 -> [w331]
    tunnel: w73 -> [_]
    shift-right: [w324] -> _
    shift-left: w78 -> [w326]
    shift-right: [w325] -> _
    shift-left: w75 -> [w327]
    shift-right: [w323] -> _
    shift-left: w82 -> [w321]
    shift-right: [w322] -> _
    shift-left: w81 -> [w320]
    stop <- w336 stop-if-true
    # "Centre Stand"
    n129 = case shown="\"Setup\"" "Centre Stand" {
      tunnel: w335 -> [w375 w431]
      tunnel: [w337 w426] -> w334
      tunnel: w332 -> [w365 w417]
      tunnel: w331 -> [w367 w420]
      tunnel: [w365 w417] -> w330
      tunnel: [w366 w418] -> w329
      tunnel: w326 -> [w349 w396]
      tunnel: w327 -> [w355 w399]
      tunnel: [w350 w397] -> w325
      tunnel: [w349 w396] -> w324
      tunnel: w321 -> [w342 w395]
      tunnel: w320 -> [w341 w393]
      tunnel: [w338 w394] -> w322
      tunnel: [w342 w395] -> w323
      frame "Main", Default {
        n130 = xnode "Read/Write Control"("FPGA VI Reference In"=w375) -> ("FPGA VI Reference Out"=w374:refnum<k20>)  [unwired: 1 in, 2 out]
        n131 = Delete From Array(array=w355, length=1, index=0) -> (array with subset deleted=w356:dbl[])  [unwired: 1 out]
        n132 = Delete From Array(array=w341, length=1, index=0) -> (array with subset deleted=w346:dbl[])  [unwired: 1 out]
        n133 = Delete From Array(array=w367, length=1, index=0) -> (array with subset deleted=w370:dbl[])  [unwired: 1 out]
        n134 = xnode "Read/Write Control"("FPGA VI Reference In"=w374) -> ("FPGA VI Reference Out"=w373:refnum<k20>)  [unwired: 1 in, 2 out]
        n135 = xnode "Read/Write Control"("FPGA VI Reference In"=w373) -> ("FPGA VI Reference Out"=w372:refnum<k20>, "Data"=w361:i32)  [unwired: 1 in, 1 out]
        n136 = Build Array (concatenate)(w370, w361) -> (w366:dbl[])
        n137 = property on="Centre LC1 zero point" class="DigNum (strict)"() -> ("Value"=w362:i32)  [unwired: 2 in, 2 out]
        n138 = property on="Centre LC2 zero point" class="DigNum (strict)"() -> ("Value"=w352:i32)  [unwired: 2 in, 2 out]
        n139 = Subtract(x=w361, y=w362) -> (x-y=w363:i32)
        n140 = property on="Centre LC1 Calibration Constant" class="DigNum (strict)"() -> ("Value"=w364:dbl)  [unwired: 2 in, 2 out]
        n141 = property on="Centre LC3 zero point" class="DigNum (strict)"() -> ("Value"=w348:i32)  [unwired: 2 in, 2 out]
        n142 = property on="Centre LC2 Calibration Constant" class="DigNum (strict)"() -> ("Value"=w353:dbl)  [unwired: 2 in, 2 out]
        n143 = xnode "Read/Write Control"("FPGA VI Reference In"=w372) -> ("FPGA VI Reference Out"=w371:refnum<k20>, "Data 2"=w351:i32)  [unwired: 1 in, 1 out]
        n144 = Build Array (concatenate)(w356, w351) -> (w350:dbl[])
        n145 = Subtract(x=w351, y=w352) -> (x-y=w359:i32)
        n146 = property on="Centre LC3 Calibration Constant" class="DigNum (strict)"() -> ("Value"=w347:dbl)  [unwired: 2 in, 2 out]
        n147 = Multiply(x=w364, y=w363) -> (x*y=→"Right LC1":dbl)
        n148 = Multiply(x=w353, y=w359) -> (x*y=→"Left LC2":dbl)
        n149 = xnode "Read/Write Control"("FPGA VI Reference In"=w371) -> ("FPGA VI Reference Out"=w337:refnum<k20>, "Data 3"=w339:i32)  [unwired: 1 in, 1 out]
        n150 = Build Array (concatenate)(w346, w339) -> (w338:dbl[])
        n151 = Subtract(x=w339, y=w348) -> (x-y=w343:i32)
        n152 = Multiply(x=w347, y=w343) -> (x*y=→"Centre LC3":dbl)
      }
      frame "Setup" {
        n153 = xnode "Read/Write Control"("FPGA VI Reference In"=w431) -> ("FPGA VI Reference Out"=w430:refnum<k20>)  [unwired: 1 in, 2 out]
        n154 = Delete From Array(array=w420, length=1, index=0) -> (array with subset deleted=w419:dbl[])  [unwired: 1 out]
        n155 = Delete From Array(array=w393, length=1, index=0) -> (array with subset deleted=w389:dbl[])  [unwired: 1 out]
        n156 = Delete From Array(array=w399, length=1, index=0) -> (array with subset deleted=w403:dbl[])  [unwired: 1 out]
        n157 = xnode "Read/Write Control"("FPGA VI Reference In"=w430) -> ("FPGA VI Reference Out"=w429:refnum<k20>)  [unwired: 1 in, 2 out]
        n158 = xnode "Read/Write Control"("FPGA VI Reference In"=w429) -> ("FPGA VI Reference Out"=w428:refnum<k20>, "Data"=w410:i32)  [unwired: 1 in, 1 out]
        "Centre LC1 Reading" <- w410
        n159 = Build Array (concatenate)(w419, w410) -> (w418:dbl[])
        n160 = call-poly <vilib>:"Mean.vi"("X"=w418) -> ("mean"=w415:dbl)  [unwired: 1 out]
        n161 = Select(t=FALSE, s="Centre LC1 Calibrate", f="Centre LC1 Calibrate") -> (s? t:f=w413:bool)
        n162 = Select(t=FALSE, s="Centre LC3 Calibrate", f="Centre LC3 Calibrate") -> (s? t:f=w377:bool)
        n163 = Select(t=FALSE, s="Centre LC2 Calibrate", f="Centre LC2 Calibrate") -> (s? t:f=w380:bool)
        n164 = Select(t=FALSE, s="Centre LC1 Tare", f="Centre LC1 Tare") -> (s? t:f=w425:bool)
        n165 = Select(t=FALSE, s="Centre LC3 Tare", f="Centre LC3 Tare") -> (s? t:f=w376:bool)
        n166 = Select(t=FALSE, s="Centre LC2 Tare", f="Centre LC2 Tare") -> (s? t:f=w382:bool)
        n167 = property on="Centre LC1 Tare" class="Bool (strict)"("Value"=w425) -> ()  [unwired: 2 in, 2 out]
        n168 = property on="Centre LC3 Calibrate" class="Bool (strict)"("Value"=w377) -> ()  [unwired: 2 in, 2 out]
        n169 = property on="Centre LC2 Calibrate" class="Bool (strict)"("Value"=w380) -> ()  [unwired: 2 in, 2 out]
        n170 = property on="Centre LC2 Tare" class="Bool (strict)"("Value"=w382) -> ()  [unwired: 2 in, 2 out]
        n171 = property on="Centre LC1 Calibrate" class="Bool (strict)"("Value"=w413) -> ()  [unwired: 2 in, 2 out]
        n172 = property on="Centre LC3 Tare" class="Bool (strict)"("Value"=w376) -> ()  [unwired: 2 in, 2 out]
        n173 = xnode "Read/Write Control"("FPGA VI Reference In"=w428) -> ("FPGA VI Reference Out"=w427:refnum<k20>, "Data 2"=w398:i32)  [unwired: 1 in, 1 out]
        "Centre LC2 Reading" <- w398
        n174 = Build Array (concatenate)(w403, w398) -> (w397:dbl[])
        n175 = call-poly <vilib>:"Mean.vi"("X"=w397) -> ("mean"=w405:dbl)  [unwired: 1 out]
        n176 = case shown="True" "Centre LC1 Tare" {
          tunnel: w415 -> [_ w458]
          tunnel: [FALSE TRUE] -> w412
          tunnel: [_ w456] -> _
          frame False {
          }
          frame True {
            n177 = property on="Centre LC1 zero point" class="DigNum (strict)"("Val(Sgnl)"=w458) -> (error out=w456:errorcluster)  [unwired: 2 in, 1 out]
          }
        }
        n178 = Or(x=w412, y="Centre LC1 Calibrate") -> (x .or. y?=w414:bool)
        n179 = case shown="True" "Centre LC2 Tare" {
          tunnel: w405 -> [_ w449]
          tunnel: [FALSE TRUE] -> w407
          tunnel: [_ w447] -> _
          frame False {
          }
          frame True {
            n180 = property on="Centre LC2 zero point" class="DigNum (strict)"("Val(Sgnl)"=w449) -> (error out=w447:errorcluster)  [unwired: 2 in, 1 out]
          }
        }
        n181 = Or(x=w407, y="Centre LC2 Calibrate") -> (x .or. y?=w406:bool)
        n182 = case shown="True" w414 {
          tunnel: w415 -> [_ w454]
          frame False {
          }
          frame True {
            n183 = local read "Centre LC1 zero point"() -> (w453:i32)
            n184 = Subtract(x=w454, y=w453) -> (x-y=w452:dbl)
            n185 = Divide(x="Centre LC1 Calibration Weight (kg)", y=w452) -> (x/y=→"Centre LC1 Calibration Constant":dbl)
          }
        }
        n186 = case shown="True" w406 {
          tunnel: w405 -> [_ w445]
          frame False {
          }
          frame True {
            n187 = local read "Centre LC2 zero point"() -> (w444:i32)
            n188 = Subtract(x=w445, y=w444) -> (x-y=w443:dbl)
            n189 = Divide(x="Centre LC2 Calibration Weight (kg)", y=w443) -> (x/y=→"Centre LC2 Calibration Constant":dbl)
          }
        }
        n190 = xnode "Read/Write Control"("FPGA VI Reference In"=w427) -> ("FPGA VI Reference Out"=w426:refnum<k20>, "Data 3"=w384:i32)  [unwired: 1 in, 1 out]
        "Centre LC3 Reading" <- w384
        n191 = Build Array (concatenate)(w389, w384) -> (w394:dbl[])
        n192 = call-poly <vilib>:"Mean.vi"("X"=w394) -> ("mean"=w387:dbl)  [unwired: 1 out]
        n193 = case shown="True" "Centre LC3 Tare" {
          tunnel: w387 -> [_ w440]
          tunnel: [FALSE TRUE] -> w385
          tunnel: [_ w438] -> _
          frame False {
          }
          frame True {
            n194 = property on="Centre LC3 zero point" class="DigNum (strict)"("Val(Sgnl)"=w440) -> (error out=w438:errorcluster)  [unwired: 2 in, 1 out]
          }
        }
        n195 = Or(x=w385, y="Centre LC3 Calibrate") -> (x .or. y?=w386:bool)
        n196 = case shown="True" w386 {
          tunnel: w387 -> [_ w436]
          frame False {
          }
          frame True {
            n197 = local read "Centre LC3 zero point"() -> (w435:i32)
            n198 = Subtract(x=w436, y=w435) -> (x-y=w434:dbl)
            n199 = Divide(x="Centre LC3 Calibration Weight (kg)", y=w434) -> (x/y=→"Centre LC3 Calibration Constant":dbl)
          }
        }
        n200 = Bundle(cluster=cluster{"Data":i32, "Data 2":i32, "Data 3":i32} {"Data"=0, "Data 2"=0, "Data 3"=0}, "Data"=w410, "Data 2"=w398, "Data 3"=w384) -> (→"Centre Raw Load Cell Readings":cluster{"Data":i32, "Data 2":i32, "Data 3":i32})
      }
    }
    n201 = Wait (ms)(milliseconds to wait=u32 20) -> ()  [unwired: 1 out]
    n202 = local read "StopLoops"() -> (w336:bool)
  }
  n203 = flat-sequence {
    tunnel: [w459] -> w37
    tunnel: [w462] -> w8
    tunnel: w37 -> [w462]
    tunnel: [w461] -> _
    frame #0 {
      n204 = call <userlib>:"port Handler.vi"("port_name"="COM3") -> ("function return"=w459:i32)  [unwired: 9 in, 1 out]
      "function return" <- w459
    }
    frame #1 {
      n205 = call <userlib>:"packet Handler.vi"() -> ("error out"=w461:errorcluster)  [unwired: 11 in]
    }
  }
  n206 = flat-sequence {
    tunnel: w8 -> [w466]
    tunnel: [w464] -> w36
    frame #0 {
      n207 = call <userlib>:"open Port.vi"("port_num"=w466) -> ("error out"=w465:errorcluster)  [unwired: 9 in, 1 out]
      n208 = call <userlib>:"set Baud Rate.vi"("error in (no error)"=w465, "baudrate"=57600, "port_num"=w466) -> ("error out"=w464:errorcluster)  [unwired: 7 in, 1 out]
    }
  }
  n209 = call <userlib>:"write1Byte Tx Rx.vi"("data"=u32 1, "address"=u16 64, "error in (no error)"=w36, "id"=u8 1, "protocol_version"=2, "port_num"=w8) -> ("error out"=w16:errorcluster)  [unwired: 5 in]
  n210 = call <userlib>:"write1Byte Tx Rx.vi"("data"=u32 1, "address"=u16 64, "error in (no error)"=w16, "id"=u8 2, "protocol_version"=2, "port_num"=w8) -> ("error out"=w15:errorcluster)  [unwired: 5 in]
  n211 = call <userlib>:"write4Byte Tx Rx.vi"("data"="Motor 1 Operating Mode", "address"=u16 11, "error in (no error)"=w15, "id"=u8 1, "protocol_version"=2, "port_num"=w8) -> ("error out"=w10:errorcluster)  [unwired: 5 in]
  n212 = xnode "Invoke Method"("FPGA VI Reference In"=w68) -> ("FPGA VI Reference Out"=w83:refnum<k20>)  [unwired: 1 in, 1 out]
  n213 = call <userlib>:"write4Byte Tx Rx.vi"("data"="Motor 2 Operating Mode", "address"=u16 11, "error in (no error)"=w10, "id"=u8 2, "protocol_version"=2, "port_num"=w8) -> ("error out"=w9:errorcluster)  [unwired: 5 in]
  n214 = xnode "Close FPGA VI Reference"("FPGA VI Reference In"=w83) -> ()  [unwired: 1 in, 1 out]
  n215 = while {
    tunnel: w8 -> [w492]
    shift-right: [w475] -> w23
    shift-left: w9 -> [w510]
    shift-right: [w501] -> _
    shift-left: u32 0 ("milliseconds to wait") -> [w503]
    tunnel: [w470] -> w3
    shift-right: [w480] -> _
    shift-left: u32 0 ("milliseconds to wait") -> [w482]
    stop <- w493 stop-if-true
    # "Motor 1"
    # "Motor 2"
    # "Get Position"
    # "Motor 2"
    # "Motor 1"
    # "Get Position"
    # "0-4095 = 0-360"
    # "Dynamixel Motors"
    n216 = Divide(x=4096.0 ("y"), y=360.0 ("x")) -> (x/y=w497:dbl)
    n217 = Multiply(x="Target Motor 1 Position", y=w497) -> (x*y=w504:dbl)
    n218 = To Word Integer(number=w504) -> (16bit integer=w500:i16)
    n219 = Not Equal?(x=w503, y=w500) -> (x != y?=w502:bool)
    n220 = Divide(x=4096.0 ("y"), y=360.0 ("x")) -> (x/y=w491:dbl)
    n221 = Multiply(x="Target Motor 2 Position", y=w491) -> (x*y=w488:dbl)
    n222 = Wait (ms)(milliseconds to wait=u32 10) -> ()  [unwired: 1 out]
    n223 = case shown="True" w502 {
      tunnel: w510 -> [w523 w527]
      tunnel: [w523 w526] -> w484
      tunnel: w492 -> [w521 w524]
      tunnel: w503 -> [w522 _]
      tunnel: [w522 w525] -> w501
      tunnel: w500 -> [_ w525]
      tunnel: [w521 w524] -> w485
      frame False {
      }
      frame True {
        # "Set Position"
        n224 = call <userlib>:"write4Byte Tx Rx.vi"("data"=w525, "address"=u16 116, "error in (no error)"=w527, "id"=u8 1, "protocol_version"=2, "port_num"=w524) -> ("error out"=w526:errorcluster)  [unwired: 5 in]
      }
    }
    n225 = To Word Integer(number=w488) -> (16bit integer=w481:i16)
    n226 = Not Equal?(x=w482, y=w481) -> (x != y?=w487:bool)
    n227 = case shown="True" w487 {
      tunnel: w484 -> [w513 w514]
      tunnel: [w513 w517] -> w483
      tunnel: w482 -> [w512 _]
      tunnel: [w512 w516] -> w480
      tunnel: w481 -> [_ w516]
      tunnel: [w511 w515] -> w470
      tunnel: w485 -> [w511 w515]
      frame False {
      }
      frame True {
        # "Set Position"
        n228 = call <userlib>:"write4Byte Tx Rx.vi"("data"=w516, "address"=u16 116, "error in (no error)"=w514, "id"=u8 2, "protocol_version"=2, "port_num"=w515) -> ("error out"=w517:errorcluster)  [unwired: 5 in]
      }
    }
    n229 = call <userlib>:"read4Byte Tx Rx.vi"("address"=u16 132, "error in (no error)"=w483, "id"=u8 1, "protocol_version"=2, "port_num"=w470) -> ("error out"=w476:errorcluster, "function return"=w505:u32)  [unwired: 5 in]
    n230 = Divide(x=4096.0, y=360.0) -> (x/y=w506:dbl)
    n231 = Divide(x=w505, y=w506) -> (x/y=→"Current Motor 1 Position":dbl)
    n232 = call <userlib>:"read4Byte Tx Rx.vi"("address"=u16 132, "error in (no error)"=w476, "id"=u8 2, "protocol_version"=2, "port_num"=w470) -> ("error out"=w475:errorcluster, "function return"=w469:u32)  [unwired: 5 in]
    n233 = Divide(x=4096.0, y=360.0) -> (x/y=w472:dbl)
    n234 = Divide(x=w469, y=w472) -> (x/y=→"Current Motor 2 Position":dbl)
    n235 = local read "StopLoops"() -> (w493:bool)
  }
  n236 = xnode "Open FPGA VI Reference"() -> ("FPGA VI Reference Out"=w111:refnum<k20>)  [unwired: 2 in, 1 out]
  n237 = property on="Right LC1 Calibration Constant" class="DigNum (strict)"("Value"=-0.5952380952379921 ("Right LC1 Calibration Constant")) -> (error out=w96:errorcluster)  [unwired: 2 in, 1 out]
  n238 = invoke on="Right PWM pulse width" class="DigNum (strict)" method="Reinit To Default"() -> (error out=w101:errorcluster)  [unwired: 3 in, 2 out]
  n239 = xnode "Invoke Method"("FPGA VI Reference In"=w111) -> ("FPGA VI Reference Out"=w110:refnum<k20>)  [unwired: 2 in, 1 out]
  n240 = Initialize Array(0.0 ("element"), 10 ("dimension size")) -> (w98:dbl[])
  n241 = Initialize Array(0.0 ("element"), 10 ("dimension size")) -> (w94:dbl[])
  n242 = Initialize Array(0.0 ("element"), 10 ("dimension size")) -> (w104:dbl[])
  n243 = Initialize Array(0.0 ("element"), 100 ("dimension size")) -> (w85:dbl[])
  n244 = Initialize Array(0.0 ("element"), 100 ("dimension size")) -> (w105:dbl[])
  n245 = Initialize Array(0.0 ("element"), 100 ("dimension size")) -> (w91:dbl[])
  n246 = while {
    tunnel: w110 -> [w552]
    tunnel: [w551] -> w108
    shift-right: [w547] -> _
    shift-left: w97 -> [w549]
    shift-right: [w546] -> _
    shift-left: w105 -> [w548]
    shift-right: [w543] -> _
    shift-left: w104 -> [w544]
    tunnel: w101 -> [_]
    shift-right: [w541] -> _
    shift-left: w98 -> [w542]
    tunnel: w96 -> [_]
    shift-right: [w539] -> _
    shift-left: w94 -> [w540]
    shift-right: [w535] -> _
    shift-left: w88 -> [w537]
    shift-right: [w536] -> _
    shift-left: w91 -> [w538]
    shift-right: [w534] -> _
    shift-left: w84 -> [w532]
    shift-right: [w533] -> _
    shift-left: w85 -> [w531]
    stop <- w553 stop-if-true
    # "Right Stand"
    n247 = case shown="\"Setup\"" "Right Stand" {
      tunnel: w552 -> [w638 w706]
      tunnel: [w585 w701] -> w551
      tunnel: w549 -> [w628 w692]
      tunnel: w548 -> [w630 w695]
      tunnel: [w628 w692] -> w547
      tunnel: [w629 w693] -> w546
      tunnel: w544 -> [w613 w685]
      tunnel: [w612 w685] -> w543
      tunnel: w542 -> [w593 w684]
      tunnel: [w588 w684] -> w541
      tunnel: w540 -> [w579 w680]
      tunnel: [w576 w680] -> w539
      tunnel: w537 -> [w565 w668]
      tunnel: w538 -> [w571 w671]
      tunnel: [w566 w669] -> w536
      tunnel: [w565 w668] -> w535
      tunnel: w532 -> [w558 w667]
      tunnel: w531 -> [w557 w665]
      tunnel: [w554 w666] -> w533
      tunnel: [w558 w667] -> w534
      frame "Main", Default {
        n248 = xnode "Read/Write Control"("FPGA VI Reference In"=w638) -> ("FPGA VI Reference Out"=w637:refnum<k20>, "RawVoltage"=w610:i16)  [unwired: 1 in, 1 out]
        n249 = Delete From Array(array=w571, length=1, index=0) -> (array with subset deleted=w572:dbl[])  [unwired: 1 out]
        n250 = Delete From Array(array=w557, length=1, index=0) -> (array with subset deleted=w562:dbl[])  [unwired: 1 out]
        n251 = Delete From Array(array=w593, length=1, index=0) -> (array with subset deleted=w592:dbl[])  [unwired: 1 out]
        n252 = Delete From Array(array=w613, length=1, index=0) -> (array with subset deleted=w619:dbl[])  [unwired: 1 out]
        n253 = Delete From Array(array=w630, length=1, index=0) -> (array with subset deleted=w633:dbl[])  [unwired: 1 out]
        n254 = xnode "Read/Write Control"("FPGA VI Reference In"=w637) -> ("FPGA VI Reference Out"=w636:refnum<k20>, "RawCurrent"=w589:u16)  [unwired: 1 in, 1 out]
        n255 = Build Array (concatenate)(w592, w589) -> (w588:dbl[])
        n256 = Build Array (concatenate)(w619, w610) -> (w612:dbl[])
        n257 = call-poly <vilib>:"Mean.vi"("X"=w588) -> ("mean"=w587:dbl)  [unwired: 1 out]
        n258 = call-poly <vilib>:"Mean.vi"("X"=w612) -> ("mean"=w617:dbl)  [unwired: 1 out]
        n259 = Divide(x=i16 20, y=i16 4096) -> (x/y=w618:dbl)
        n260 = Multiply(x=w617, y=w618) -> (x*y=w615:dbl)
        n261 = xnode "Read/Write Control"("FPGA VI Reference In"=w636) -> ("FPGA VI Reference Out"=w635:refnum<k20>, "Data"=w624:i32)  [unwired: 1 in, 1 out]
        n262 = Build Array (concatenate)(w633, w624) -> (w629:dbl[])
        n263 = property on="Right LC1 zero point" class="DigNum (strict)"() -> ("Value"=w625:i32)  [unwired: 2 in, 2 out]
        n264 = Add(x="Right Resistance Vout (Ohms)", y="Right Resistance non-Vout (Ohms)") -> (x+y=w609:dbl)
        n265 = property on="Right LC2 zero point" class="DigNum (strict)"() -> ("Value"=w568:i32)  [unwired: 2 in, 2 out]
        n266 = Subtract(x=w624, y=w625) -> (x-y=w626:i32)
        n267 = property on="Right LC1 Calibration Constant" class="DigNum (strict)"() -> ("Value"=w627:dbl)  [unwired: 2 in, 2 out]
        n268 = property on="Right LC3 zero point" class="DigNum (strict)"() -> ("Value"=w564:i32)  [unwired: 2 in, 2 out]
        n269 = property on="Right LC2 Calibration Constant" class="DigNum (strict)"() -> ("Value"=w569:dbl)  [unwired: 2 in, 2 out]
        n270 = xnode "Read/Write Control"("FPGA VI Reference In"=w635) -> ("FPGA VI Reference Out"=w634:refnum<k20>, "Data 2"=w567:i32)  [unwired: 1 in, 1 out]
        n271 = Build Array (concatenate)(w572, w567) -> (w566:dbl[])
        n272 = Subtract(x=w567, y=w568) -> (x-y=w575:i32)
        n273 = property on="Right LC3 Calibration Constant" class="DigNum (strict)"() -> ("Value"=w563:dbl)  [unwired: 2 in, 2 out]
        n274 = Divide(x=w609, y="Right Resistance Vout (Ohms)") -> (x/y=w614:dbl)
        n275 = Multiply(x=w614, y=w615) -> (x*y=→"Right Voltage":dbl)
        n276 = Divide(x=i16 5, y=i16 4096) -> (x/y=w605:dbl)
        n277 = Multiply(x=w627, y=w626) -> (x*y=→"Right LC1":dbl)
        n278 = Multiply(x=w569, y=w575) -> (x*y=→"Right LC2":dbl)
        n279 = Multiply(x=w587, y=w605) -> (x*y=w595:dbl)
        n280 = Divide(x=i16 90 ("y"), y=3.3 ("x")) -> (x/y=w604:dbl)
        n281 = xnode "Read/Write Control"("FPGA VI Reference In"=w634) -> ("FPGA VI Reference Out"=w603:refnum<k20>, "Data 3"=w555:i32)  [unwired: 1 in, 1 out]
        n282 = Build Array (concatenate)(w562, w555) -> (w554:dbl[])
        n283 = Subtract(x=w555, y=w564) -> (x-y=w559:i32)
        n284 = Multiply(x=w563, y=w559) -> (x*y=→"Right LC3":dbl)
        n285 = Multiply(x=w595, y=w604) -> (x*y=→"Right Current":dbl)
        n286 = xnode "Read/Write Control"("FPGA VI Reference In"=w603, "Pulse Width (us)"="Right PWM pulse width") -> ("FPGA VI Reference Out"=w601:refnum<k20>)  [unwired: 1 in, 1 out]
        n287 = xnode "Read/Write Control"("FPGA VI Reference In"=w601, "Frequency"="Right PWM frequency") -> ("FPGA VI Reference Out"=w599:refnum<k20>)  [unwired: 1 in, 1 out]
        n288 = xnode "Read/Write Control"("FPGA VI Reference In"=w599, "PWM Switch"="Right PWM Switch") -> ("FPGA VI Reference Out"=w598:refnum<k20>)  [unwired: 1 in, 1 out]
        n289 = xnode "Read/Write Control"("FPGA VI Reference In"=w598) -> ("FPGA VI Reference Out"=w585:refnum<k20>, "Rotor Speed (Hz)"=w583:sgl)  [unwired: 1 in, 1 out]
        n290 = case shown="True" "Right PWM Switch" {
          tunnel: [0.0 ("Motor Frequency") w641] -> w578
          tunnel: w583 -> [_ w640]
          frame False {
          }
          frame True {
            w647 = T1 1 items=["RPM", "Hz"] ("Right Motor Units")
            n291 = Equal?(x="Right Motor Units", y=w647) -> (x = y?=w646:bool)
            n292 = Select(t=1.0, s=w646, f=60.0) -> (s? t:f=w642:dbl)
            n293 = Multiply(x=w642, y=w640) -> (x*y=w641:dbl)
          }
        }
        n294 = Delete From Array(array=w579, length=1, index=0) -> (array with subset deleted=w580:dbl[])  [unwired: 1 out]
        n295 = Build Array (concatenate)(w580, w578) -> (w576:dbl[])
        n296 = call-poly <vilib>:"Mean.vi"("X"=w576) -> ("mean"=→"Right Motor Frequency":dbl)  [unwired: 1 out]
      }
      frame "Setup" {
        n297 = xnode "Read/Write Control"("FPGA VI Reference In"=w706) -> ("FPGA VI Reference Out"=w705:refnum<k20>)  [unwired: 1 in, 2 out]
        n298 = Delete From Array(array=w695, length=1, index=0) -> (array with subset deleted=w694:dbl[])  [unwired: 1 out]
        n299 = Delete From Array(array=w665, length=1, index=0) -> (array with subset deleted=w661:dbl[])  [unwired: 1 out]
        n300 = Delete From Array(array=w671, length=1, index=0) -> (array with subset deleted=w675:dbl[])  [unwired: 1 out]
        n301 = xnode "Read/Write Control"("FPGA VI Reference In"=w705) -> ("FPGA VI Reference Out"=w704:refnum<k20>)  [unwired: 1 in, 2 out]
        n302 = xnode "Read/Write Control"("FPGA VI Reference In"=w704) -> ("FPGA VI Reference Out"=w703:refnum<k20>, "Data"=w683:i32)  [unwired: 1 in, 1 out]
        "Right LC1 Reading" <- w683
        n303 = Build Array (concatenate)(w694, w683) -> (w693:dbl[])
        n304 = call-poly <vilib>:"Mean.vi"("X"=w693) -> ("mean"=w690:dbl)  [unwired: 1 out]
        n305 = Select(t=FALSE, s="Right LC1 Calibrate", f="Right LC1 Calibrate") -> (s? t:f=w688:bool)
        n306 = Select(t=FALSE, s="Right LC3 Calibrate", f="Right LC3 Calibrate") -> (s? t:f=w649:bool)
        n307 = Select(t=FALSE, s="Right LC2 Calibrate", f="Right LC2 Calibrate") -> (s? t:f=w652:bool)
        n308 = Select(t=FALSE, s="Right LC1 Tare", f="Right LC1 Tare") -> (s? t:f=w700:bool)
        n309 = Select(t=FALSE, s="Right LC3 Tare", f="Right LC3 Tare") -> (s? t:f=w648:bool)
        n310 = Select(t=FALSE, s="Right LC2 Tare", f="Right LC2 Tare") -> (s? t:f=w654:bool)
        n311 = property on="Right LC1 Tare" class="Bool (strict)"("Value"=w700) -> ()  [unwired: 2 in, 2 out]
        n312 = property on="Right LC3 Calibrate" class="Bool (strict)"("Value"=w649) -> ()  [unwired: 2 in, 2 out]
        n313 = property on="Right LC2 Calibrate" class="Bool (strict)"("Value"=w652) -> ()  [unwired: 2 in, 2 out]
        n314 = property on="Right LC2 Tare" class="Bool (strict)"("Value"=w654) -> ()  [unwired: 2 in, 2 out]
        n315 = property on="Right LC1 Calibrate" class="Bool (strict)"("Value"=w688) -> ()  [unwired: 2 in, 2 out]
        n316 = property on="Right LC3 Tare" class="Bool (strict)"("Value"=w648) -> ()  [unwired: 2 in, 2 out]
        n317 = xnode "Read/Write Control"("FPGA VI Reference In"=w703) -> ("FPGA VI Reference Out"=w702:refnum<k20>, "Data 2"=w670:i32)  [unwired: 1 in, 1 out]
        "Right LC2 Reading" <- w670
        n318 = Build Array (concatenate)(w675, w670) -> (w669:dbl[])
        n319 = call-poly <vilib>:"Mean.vi"("X"=w669) -> ("mean"=w677:dbl)  [unwired: 1 out]
        n320 = case shown="True" "Right LC1 Tare" {
          tunnel: w690 -> [_ w733]
          tunnel: [FALSE TRUE] -> w687
          tunnel: [_ w731] -> _
          frame False {
          }
          frame True {
            n321 = property on="Right LC1 zero point" class="DigNum (strict)"("Val(Sgnl)"=w733) -> (error out=w731:errorcluster)  [unwired: 2 in, 1 out]
          }
        }
        n322 = Or(x=w687, y="Right LC1 Calibrate") -> (x .or. y?=w689:bool)
        n323 = case shown="True" "Right LC2 Tare" {
          tunnel: w677 -> [_ w724]
          tunnel: [FALSE TRUE] -> w679
          tunnel: [_ w722] -> _
          frame False {
          }
          frame True {
            n324 = property on="Right LC2 zero point" class="DigNum (strict)"("Val(Sgnl)"=w724) -> (error out=w722:errorcluster)  [unwired: 2 in, 1 out]
          }
        }
        n325 = Or(x=w679, y="Right LC2 Calibrate") -> (x .or. y?=w678:bool)
        n326 = case shown="True" w689 {
          tunnel: w690 -> [_ w729]
          frame False {
          }
          frame True {
            n327 = local read "Right LC1 zero point"() -> (w728:i32)
            n328 = Subtract(x=w729, y=w728) -> (x-y=w727:dbl)
            n329 = Divide(x="Right LC1 Calibration Weight (kg)", y=w727) -> (x/y=→"Right LC1 Calibration Constant":dbl)
          }
        }
        n330 = case shown="True" w678 {
          tunnel: w677 -> [_ w720]
          frame False {
          }
          frame True {
            n331 = local read "Right LC2 zero point"() -> (w719:i32)
            n332 = Subtract(x=w720, y=w719) -> (x-y=w718:dbl)
            n333 = Divide(x="Right LC2 Calibration Weight (kg)", y=w718) -> (x/y=→"Right LC2 Calibration Constant":dbl)
          }
        }
        n334 = xnode "Read/Write Control"("FPGA VI Reference In"=w702) -> ("FPGA VI Reference Out"=w701:refnum<k20>, "Data 3"=w656:i32)  [unwired: 1 in, 1 out]
        "Right LC3 Reading" <- w656
        n335 = Build Array (concatenate)(w661, w656) -> (w666:dbl[])
        n336 = call-poly <vilib>:"Mean.vi"("X"=w666) -> ("mean"=w659:dbl)  [unwired: 1 out]
        n337 = case shown="True" "Right LC3 Tare" {
          tunnel: w659 -> [_ w715]
          tunnel: [FALSE TRUE] -> w657
          tunnel: [_ w713] -> _
          frame False {
          }
          frame True {
            n338 = property on="Right LC3 zero point" class="DigNum (strict)"("Val(Sgnl)"=w715) -> (error out=w713:errorcluster)  [unwired: 2 in, 1 out]
          }
        }
        n339 = Or(x=w657, y="Right LC3 Calibrate") -> (x .or. y?=w658:bool)
        n340 = case shown="True" w658 {
          tunnel: w659 -> [_ w711]
          frame False {
          }
          frame True {
            n341 = local read "Right LC3 zero point"() -> (w710:i32)
            n342 = Subtract(x=w711, y=w710) -> (x-y=w709:dbl)
            n343 = Divide(x="Right LC3 Calibration Weight (kg)", y=w709) -> (x/y=→"Right LC3 Calibration Constant":dbl)
          }
        }
        n344 = Bundle(cluster=cluster{"Data":i32, "Data 2":i32, "Data 3":i32} {"Data"=0, "Data 2"=0, "Data 3"=0}, "Data"=w683, "Data 2"=w670, "Data 3"=w656) -> (→"Right Raw Load Cell Readings":cluster{"Data":i32, "Data 2":i32, "Data 3":i32})
      }
    }
    n345 = Wait (ms)(milliseconds to wait=u32 20) -> ()  [unwired: 1 out]
    n346 = local read "StopLoops"() -> (w553:bool)
  }
  n347 = call <userlib>:"write1Byte Tx Rx.vi"("data"=u32 1, "address"=u16 64, "error in (no error)"=w23, "id"=u8 1, "protocol_version"=2, "port_num"=w3) -> ("error out"=w1:errorcluster)  [unwired: 5 in]
  n348 = call <userlib>:"write1Byte Tx Rx.vi"("data"=u32 1, "address"=u16 64, "error in (no error)"=w1, "id"=u8 2, "protocol_version"=2, "port_num"=w3) -> ("error out"=w2:errorcluster)  [unwired: 5 in]
  n349 = call <userlib>:"close Port.vi"("error in (no error)"=w2, "port_num"=w3) -> ()  [unwired: 9 in, 1 out]
  n350 = xnode "Invoke Method"("FPGA VI Reference In"=w108) -> ("FPGA VI Reference Out"=w109:refnum<k20>)  [unwired: 1 in, 1 out]
  n351 = xnode "Close FPGA VI Reference"("FPGA VI Reference In"=w109) -> ()  [unwired: 1 in, 1 out]
  "Right LC1 zero point" <- w97
  "Right LC2 zero point" <- w88
  "Right LC3 zero point" <- w84
  "Centre LC1 zero point" <- w72
  "Centre LC2 zero point" <- w78
  "Centre LC3 zero point" <- w82
  "Left LC1 zero point" <- w51
  "Left LC2 zero point" <- w42
  "Left LC3 zero point" <- w38
